vi "getTemperature.vi"(8 "error in (no error)":errorcluster, 11 "CameraNetworkController in":refnum<class "CameraNetworkController.lvclass">) -> (0 "error out":errorcluster, 2 "temperature":dbl, 3 "CameraNetworkController out":refnum<class "CameraNetworkController.lvclass">)   [LabVIEW 2011, in "Hardware.lvlib" / "HWControllers.lvlib" / "CameraNetworkController.lvclass"]
uses:
  CameraNetworkController.lvclass
  NetworkClient/NetworkServer.lvclass
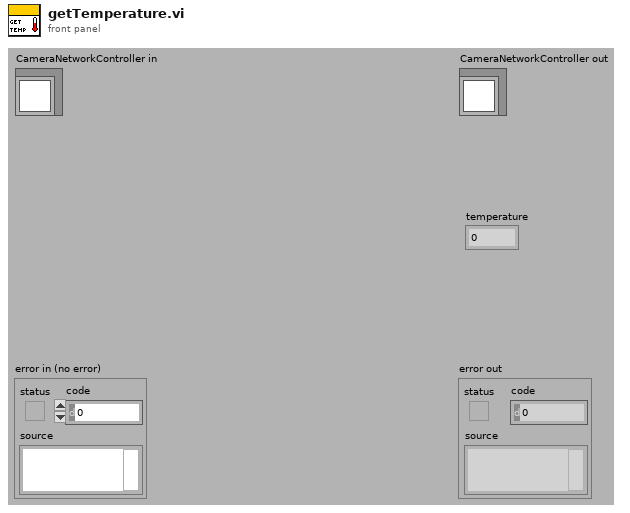
[diagram p1: front panel]
types:
  T1 = cluster{"Message":enum16{"Idle", "initialise", "configureAcquisition", "setTemperature", "getTemperature", "start", "stop", "sendImage", "close", "error", "ExitApp"}, "Data":variant}
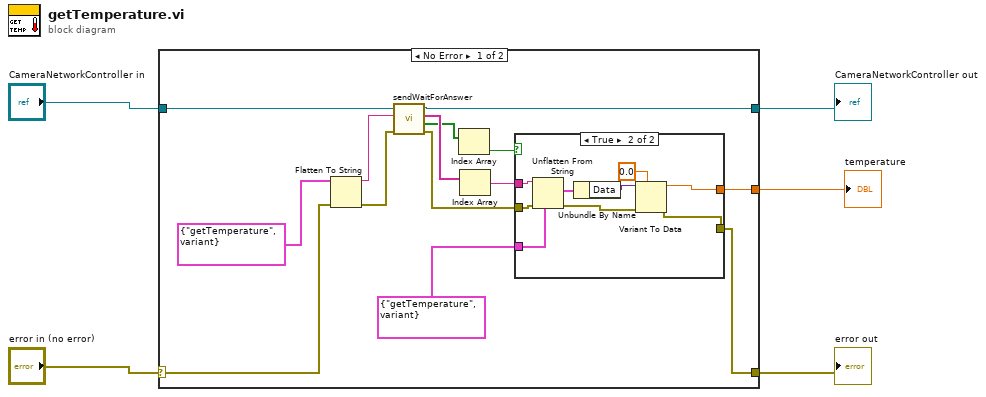
[diagram p0: block diagram]
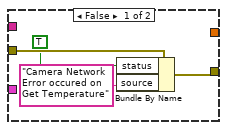
[diagram p2: hidden frame]
diagram:
  n1 = case shown="No Error" "error in (no error)" {
    selector: "error in (no error)" -> [w17 w34]
    tunnel: [w12 w34] -> w3
    tunnel: [w13 w33] -> w1
    tunnel: "CameraNetworkController in" -> [w19 w33]
    tunnel: [w6 _] -> w2
    frame No Error {
      n2 = Flatten To String(anything=T1 {"Message"=enum."getTemperature", "Data"=variant}, error in (no error)=w17) -> (data string=w18:string, error out=w10:errorcluster)  [unwired: 3 out]
      n3 = call "sendWaitForAnswer.vi"("error in (no error)"=w10, "message"=w18, "NetworkServer in"=w19) -> ("error out"=w11:errorcluster, "valid?"=w8:bool[], "answers"=w14:string[], "NetworkServer out"=w13:refnum<class "CameraNetworkController.lvclass">)  [unwired: 5 in]
      n4 = Index Array(array=w8) -> (element=w9:bool)  [unwired: 1 in]
      n5 = Index Array(array=w14) -> (element=w15:string)  [unwired: 1 in]
      n6 = case shown="True" w9 {
        tunnel: T1 {"Message"=enum."getTemperature", "Data"=variant} -> [_ w32]
        tunnel: w15 -> [_ w31]
        tunnel: [w20 w27] -> w12
        tunnel: w11 -> [w22 w25]
        tunnel: [_ w24] -> w6
        frame False {
          n7 = Bundle By Name(cluster=w22, "status"=TRUE, "source"="Camera Network Error occured on Get Temperature") -> (w20:errorcluster)
        }
        frame True {
          n8 = Unflatten From String(type=w32, binary string=w31, error in (no error)=w25) -> (value=w30:T1, error out=w26:errorcluster)  [unwired: 2 in, 1 out]
          n9 = Unbundle By Name(w30) -> ("Data"=w29:variant)
          n10 = Variant To Data(error in=w26, type=0.0, Variant=w29) -> (data=w24:dbl, error out=w27:errorcluster)
        }
      }
    }
    frame Error {
    }
  }
  "error out" <- w3
  "CameraNetworkController out" <- w1
  "temperature" <- w2
